vi "updateDB.vi"(6 "First":bool, 8 "DBname":string, 9 "Data Write":i32[](array[numeric]), 10 "Write?":bool, 11 "COM PORT":refnum<visa-resource-name>) -> (3 "DBarray":dbl[][](array[numeric]), 4 "First 2":bool)   [LabVIEW 2021]
panel:
  out "RX_DATA":i32[](array[numeric])
  out "DB_data":dbl[](array[numeric])
  out "i":i32
  out "IDs No":dbl
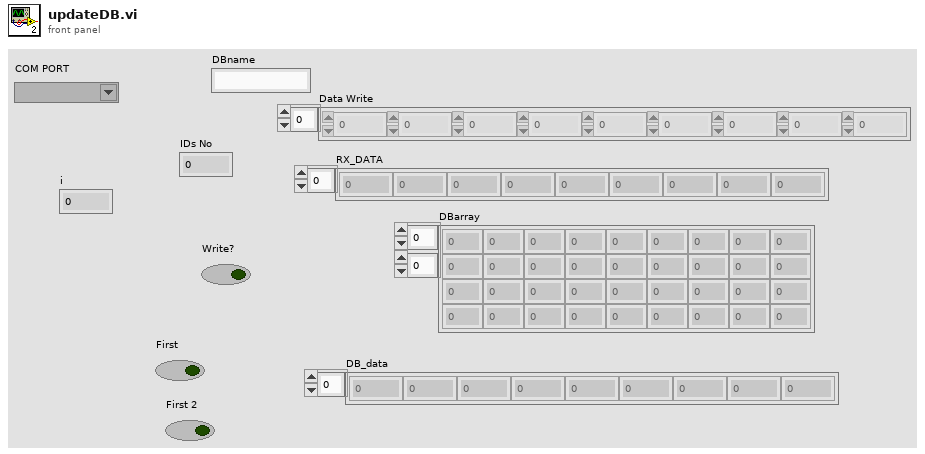
[diagram p1: front panel]
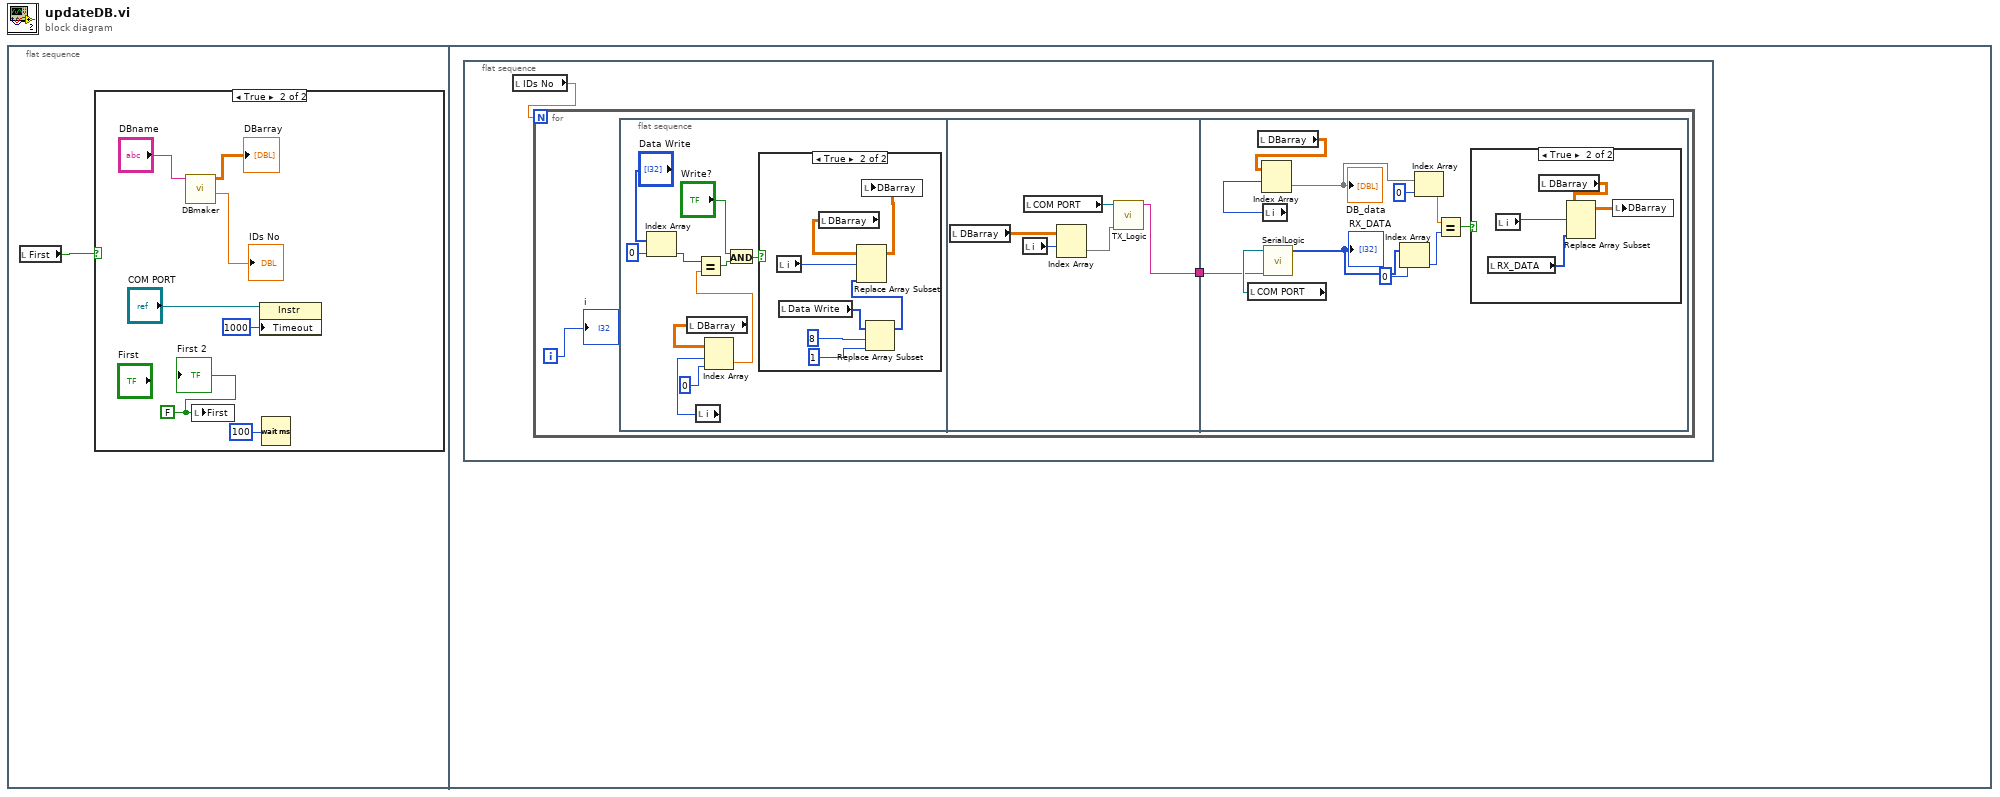
[diagram p0: block diagram]
diagram:
  n1 = flat-sequence {
    frame #0 {
      n2 = local read "First"() -> (w1:bool)
      n3 = case shown="True" w1 {
        frame False {
        }
        frame True {
          w5 = FALSE ("First")
          n4 = call "DBmaker.vi"("DBname"="DBname") -> ("IDs No"=→"IDs No":dbl, "DBarray"=→"DBarray":dbl[][])  [unwired: 7 in]
          n5 = local write "First"(w5) -> ()
          n6 = property class="Instr"(reference="COM PORT", "Timeout"=u32 1000 ("General Settings:Timeout Value")) -> ()  [unwired: 1 in, 2 out]
          n7 = Wait (ms)(milliseconds to wait=u32 100) -> ()  [unwired: 1 out]
          "First 2" <- w5
        }
      }
    }
    frame #1 {
      n8 = flat-sequence {
        frame #0 {
          n9 = local read "IDs No"() -> (w9:dbl)
          n10 = for {
            N: w9 -> [_]
            i -> [w11]
            n11 = flat-sequence {
              tunnel: [w29] -> w10
              tunnel: w10 -> [w34]
              frame #0 {
                n12 = Index Array(array="Data Write", index=0) -> (element=w12:i32)
                n13 = local read "DBarray"() -> (w19:dbl[][])
                n14 = local read "i"() -> (w18:i32)
                n15 = Index Array(array=w19, index (row)=w18, index (col)=0 ("disabled index (col)")) -> (element=w15:dbl)
                n16 = Equal?(x=w12, y=w15) -> (x = y?=w16:bool)
                n17 = And(x="Write?", y=w16) -> (x .and. y?=w21:bool)
                n18 = case shown="True" w21 {
                  frame False {
                  }
                  frame True {
                    n19 = local read "i"() -> (w26:i32)
                    n20 = local read "Data Write"() -> (w25:i32[])
                    n21 = local read "DBarray"() -> (w28:dbl[][])
                    n22 = Replace Array Subset(array=w25, new element=1 ("new element/subarray"), index=8) -> (w24:i32[])
                    n23 = Replace Array Subset(array=w28, new element=w24, index (row)=w26) -> (w27:dbl[][])  [unwired: 1 in]
                    n24 = local write "DBarray"(w27) -> ()
                  }
                }
              }
              frame #1 {
                n25 = local read "DBarray"() -> (w33:dbl[][])
                n26 = local read "i"() -> (w32:i32)
                n27 = local read "COM PORT"() -> (w31:refnum<visa-resource-name>)
                n28 = Index Array(array=w33, index (row)=w32) -> (element=w30:dbl[])  [unwired: 1 in]
                n29 = call "TX_Logic.vi"("initialized array 2"=w30, "VISA resource name"=w31) -> ("read buffer"=w29:string)  [unwired: 7 in]
              }
              frame #2 {
                n30 = local read "COM PORT"() -> (w42:refnum<visa-resource-name>)
                n31 = local read "DBarray"() -> (w44:dbl[][])
                n32 = local read "i"() -> (w43:i32)
                n33 = Index Array(array=w44, index (row)=w43) -> (element=w40:dbl[])  [unwired: 1 in]
                "DB_data" <- w40
                n34 = call "SerialLogic.vi"("read buffer"=w34, "COM PORT"=w42) -> ("RX_DATA"=w36:i32[])  [unwired: 9 in]
                "RX_DATA" <- w36
                n35 = Index Array(array=w36, index=0) -> (element=w37:i32)
                n36 = Index Array(array=w40, index=0) -> (element=w38:dbl)
                n37 = Equal?(x=w38, y=w37) -> (x = y?=w41:bool)
                n38 = case shown="True" w41 {
                  frame False {
                  }
                  frame True {
                    n39 = local read "RX_DATA"() -> (w45:i32[])
                    n40 = local read "i"() -> (w47:i32)
                    n41 = local read "DBarray"() -> (w48:dbl[][])
                    n42 = Replace Array Subset(array=w48, new element=w45, index (row)=w47) -> (w46:dbl[][])  [unwired: 1 in]
                    n43 = local write "DBarray"(w46) -> ()
                  }
                }
              }
            }
            "i" <- w11
          }
        }
      }
    }
  }
